vi "chart series set trendline forecast.vi"(8 "error in (no error)":errorcluster, 9 "backward":dbl, 10 "forward":dbl, 11 "series":u32) -> (0 "error out":errorcluster, 3 "function return":u32(ring))   [LabVIEW 2015, in "xlsxwriter.lvlib"]
doc: "lxw_error chart_series_set_trendline_forecast(lxw_chart_series series, double forward, double backward);"
uses:
  xlsxwriter.lvlib
  xlsxwriter.dll
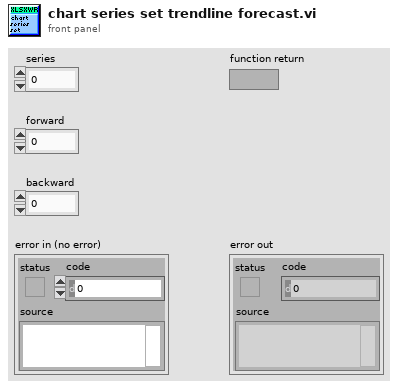
[diagram p1: front panel]
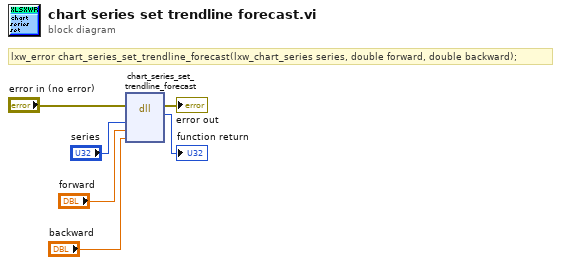
[diagram p0: block diagram]
diagram:
  # "lxw_error chart_series_set_trendline_forecast(lxw_chart_series series, double forward, double backward);"
  n1 = dll-call lib="C:/Users/WDAGUtilityAccount/Desktop/lv_vis_added_cell/xlsxwriter.*" fn="chart_series_set_trendline_forecast"(error in="error in (no error)", "series"="series", "forward"="forward", "backward"="backward") -> (error out=→"error out":errorcluster, →"function return":u32)  [unwired: 5 in, 1 out]
